vi "vision process goal.vi"(8 "Luma Range":cluster{"Lower value":i32, "Upper value":i32}={"Lower value"=40, "Upper value"=255}, 9 "Sat Range":cluster{"Lower value":i32, "Upper value":i32}={"Lower value"=52, "Upper value"=255}, 10 "Hue Range":cluster{"Lower value":i32, "Upper value":i32}={"Lower value"=80, "Upper value"=120}, 11 "Src Image":T1(plugin-control)) -> (2 "Annotated Image Out":T1(plugin-control), 3 "Processed Image Out":T1(plugin-control), 4 "Waveform Chart":dbl(graph))   [LabVIEW 2015]
uses:
  <vilib>/Rock Robotics/Network Tables/NT Read Boolean.vi
  <vilib>/Rock Robotics/Network Tables/NT Write Boolean.vi
  <vilib>/Rock Robotics/Network Tables/NT Write Number.vi
  <vilib>/vision/NI_Vision_Development_Module.lvlib
panel:
  out "output cluster":cluster{dbl[], dbl[], dbl[]}
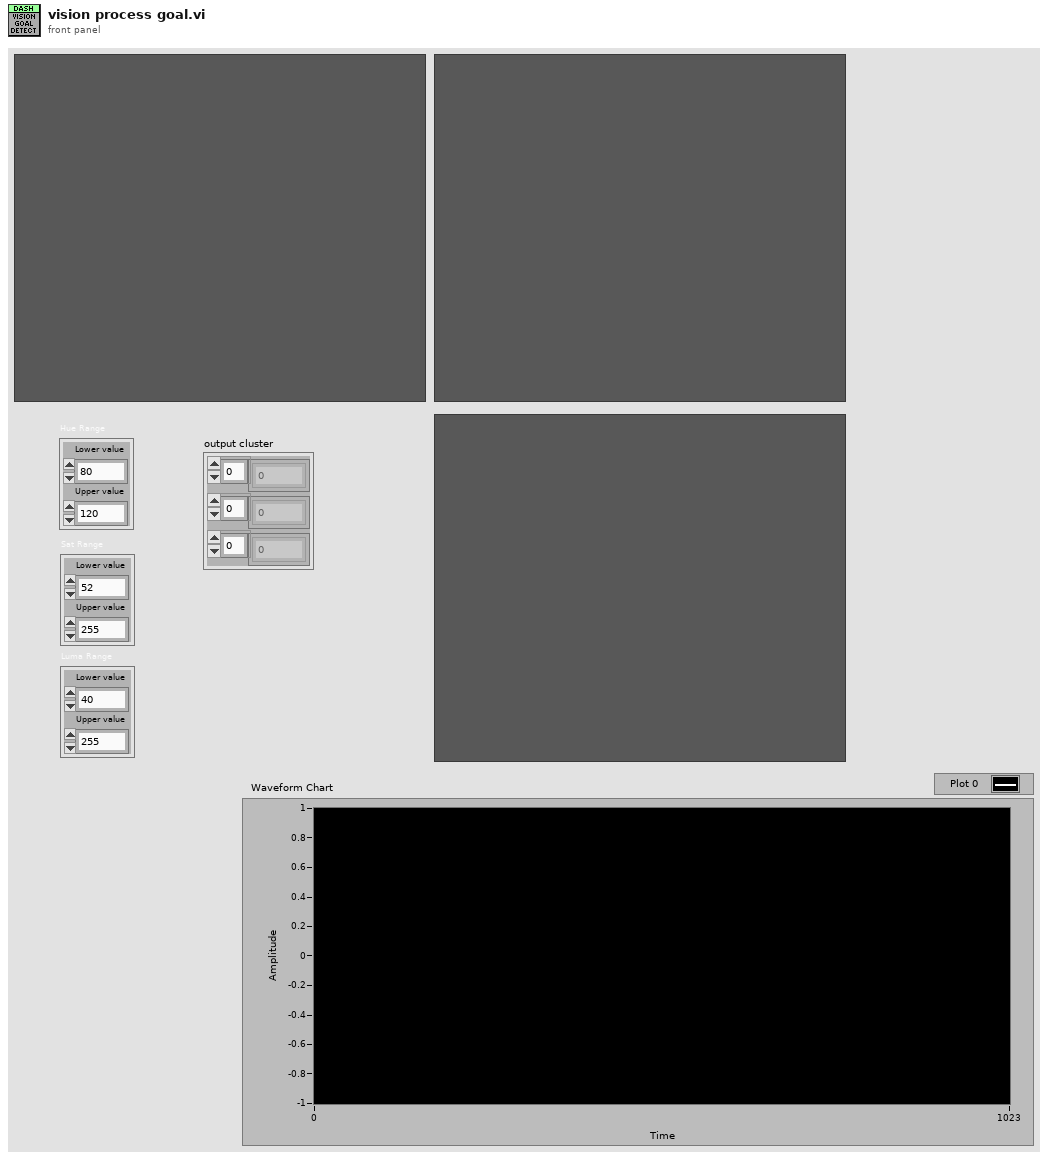
[diagram p1: front panel]
types:
  T1 = typedef "IMAQ Image.ctl" = refnum<image>
  T2 = typedef "Image Type" = u32
  T3 = cluster{"Area":dbl, "Number of Holes":dbl, "Bounding Rect":cluster{"Left":dbl, "Top":dbl, "Right":dbl, "Bottom":dbl}, "Center of Mass":cluster{"X":dbl, "Y":dbl}, "Orientation":dbl, "Dimensions":cluster{"Width":dbl, "Height":dbl}}
  T4 = cluster{"Desired Font (Application)":enum16{"User-specified Font", "Application Font", "System Font", "Dialog Font"}, "[User-specified Font]":cluster{"Font Name":string, "Size":i16, "Strikeout?":bool, "Italic?":bool, "Underline?":bool, "Outline?":bool, "Shadow?":bool, "Bold?":bool, "Rotation Angle":dbl}, "Horizontal Alignment":i16, "Vertical Alignment":i16}
  T5 = cluster{"Left":i32, "Top":i32, "Right":i32, "Bottom":i32}
  T6 = cluster{"Area":dbl, "Number of Holes":dbl, "Bounding Rect":cluster{"Left":dbl, "Top":dbl, "Right":dbl, "Bottom":dbl}, "Center of Mass":cluster{"X":dbl, "Y":dbl}, "Orientation":dbl, "Dimensions":cluster{"Width":dbl, "Height":dbl}}[]
  T7 = cluster{"Left":dbl, "Top":dbl, "Right":dbl, "Bottom":dbl}
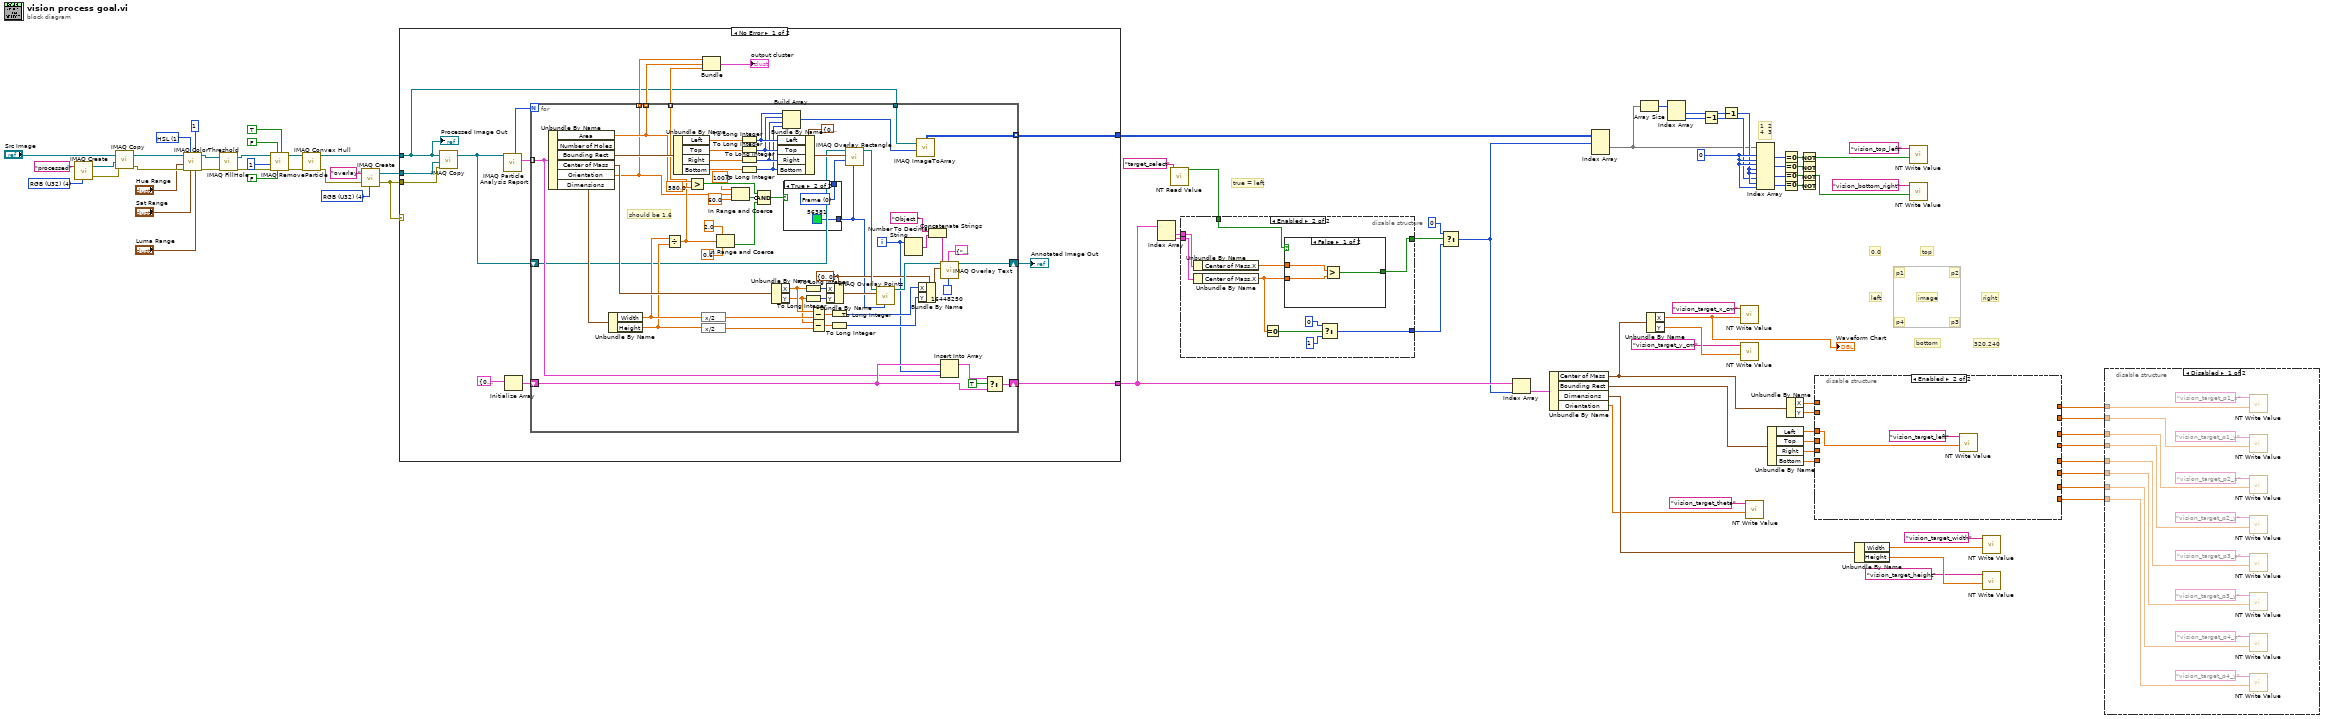
[diagram p0: block diagram]
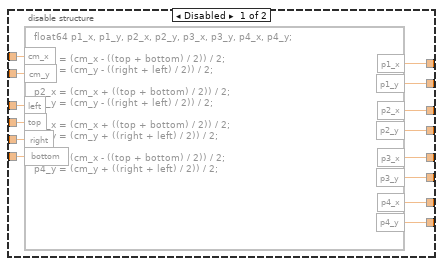
[diagram p3: hidden frame]
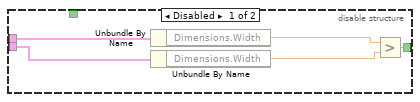
[diagram p4: hidden frame]
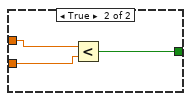
[diagram p5: hidden frame]
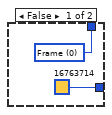
[diagram p6: hidden frame]
diagram:
  w36 = 0 ("index (row)")
  w77 = u16 1 items=["RGB", "HSL", "HSV", "HSI"] ("Color Mode")
  w79 = T2 4 items=["Grayscale (U8)", "Grayscale (I16)", "Grayscale (SGL)", "Complex (CSG)", "RGB (U32)", "HSL (U32)", "RGB (U64)", "Grayscale (U16)"] ("Image Type")
  w83 = T2 4 items=["Grayscale (U8)", "Grayscale (I16)", "Grayscale (SGL)", "Complex (CSG)", "RGB (U32)", "HSL (U32)", "RGB (U64)", "Grayscale (U16)"] ("Image Type")
  # "true = left"
  # "1  2\n4  3"
  # "320,240"
  # "0,0"
  # "top"
  # "right"
  # "left"
  # "bottom"
  # "image"
  # "p4"
  # "p3"
  # "p2"
  # "p1"
  n1 = call "IMAQ Create"("Image Name"="processed", "Image Type"=w79) -> ("New Image"=w80:T1, "error out"=w78:errorcluster)  [unwired: 3 in]
  n2 = call "IMAQ Copy"("error in (no error)"=w78, "Image Dst"=w80, "Image Src"="Src Image") -> ("error out"=w62:errorcluster, "Image Dst Out"=w73:T1)  [unwired: 3 in]
  n3 = call "IMAQ ColorThreshold"("Blue or Luma or Val or Inten Range"="Luma Range", "Replace Value"=1, "Green or Sat Range"="Sat Range", "Color Mode"=w77, "error in (no error)"=w62, "Red or Hue Range"="Hue Range", "Image Src"=w73) -> ("error out"=w63:errorcluster, "Image Dst Out"=w74:T1)  [unwired: 3 in]
  n4 = call "IMAQ FillHole"("error in (no error)"=w63, "Image Src"=w74) -> ("error out"=w64:errorcluster, "Image Dst Out"=w71:T1)  [unwired: 4 in]
  n5 = call "IMAQ RemoveParticle"("Connectivity 4/8 (8)"=TRUE, "Low Pass/High Pass (Low)"=FALSE, "Square/Hexa (Square)"=FALSE, "error in (no error)"=w64, "Number of Erosion"=1, "Image Src"=w71) -> ("error out"=w65:errorcluster, "Image Dst Out"=w66:T1)  [unwired: 1 in, 3 out]
  n6 = call "IMAQ Convex Hull"("error in (no error)"=w65, "Image Src"=w66) -> ("error out"=w58:errorcluster, "Image Dst Out"=w59:T1)  [unwired: 8 in]
  n7 = call "IMAQ Create"("Image Name"="overlay", "Image Type"=w83, "error in (no error)"=w58) -> ("New Image"=w84:T1, "error out"=w82:errorcluster)  [unwired: 2 in]
  n8 = case shown="No Error" w82 {
    tunnel: w84 -> [w97 _]
    tunnel: w59 -> [w86 _]
    tunnel: w82 -> [w96 _]
    tunnel: [w89 _] -> w12
    tunnel: [w88 _] -> w57
    frame No Error {
      n9 = call "IMAQ Copy"("error in (no error)"=w96, "Image Dst"=w97, "Image Src"=w86) -> ("Image Dst Out"=w87:T1)  [unwired: 3 in, 1 out]
      n10 = call "IMAQ Particle Analysis Report"("Image"=w87) -> ("Particle Reports (Pixels)"=w99:T6, "Number of Particles"=w100:i32)  [unwired: 5 in, 4 out]
      n11 = Initialize Array(T3 {"Area"=0.0, "Number of Holes"=0.0, "Bounding Rect"={"Left"=0.0, "Top"=0.0, "Right"=0.0, "Bottom"=0.0}, "Center of Mass"={"X"=0.0, "Y"=0.0}, "Orientation"=0.0, "Dimensions"={"Width"=0.0, "Height"=0.0}} ("Particle Report")) -> (w90:T6)  [unwired: 1 in]
      n12 = for {
        N: w100 -> [_]
        tunnel: w99 -> [w112] mode=indexing
        shift-right: [w147] -> w98
        shift-left: w87 -> [w110]
        tunnel: [w117] -> w95 mode=indexing
        tunnel: [w120] -> w94 mode=indexing
        tunnel: [w119] -> w93 mode=indexing
        shift-right: [w114] -> w89
        shift-left: w90 -> [w113]
        tunnel: [w103] -> w88 mode=indexing
        tunnel: w86 -> [w105]
        i -> [w101]
        w141 = cluster{"X":i32, "Y":i32} {"X"=0, "Y"=0} ("Point")
        # "should be 1.6"
        n13 = Unbundle By Name(w112) -> ("Area"=w120:dbl, "Bounding Rect"=w159:T7, "Center of Mass"=w153:cluster{"X":dbl, "Y":dbl}, "Orientation"=w117:dbl, "Dimensions"=w140:cluster{"Width":dbl, "Height":dbl})  [unwired: 1 out]
        n14 = Unbundle By Name(w140) -> ("Width"=w132:dbl, "Height"=w131:dbl)
        n15 = Divide(x=w132, y=w131) -> (x/y=w119:dbl)
        n16 = Unbundle By Name(w159) -> ("Left"=w157:dbl, "Top"=w156:dbl, "Right"=w155:dbl, "Bottom"=w125:dbl)
        n17 = Greater?(x=w120, y=580.0) -> (0:w123:bool)
        n18 = expression code="x/2"(w132) -> (w139:dbl)
        n19 = expression code="x/2"(w131) -> (w135:dbl)
        n20 = In Range and Coerce(upper limit=2.0, x=w119, lower limit=0.6 ("upper limit")) -> (In Range?=w128:bool)  [unwired: 1 out]
        n21 = In Range and Coerce(upper limit=100.0, x=w117, lower limit=60.0 ("y")) -> (In Range?=w118:bool)  [unwired: 1 out]
        n22 = To Long Integer(number=w157) -> (32bit integer=w109:i32)
        n23 = To Long Integer(number=w156) -> (32bit integer=w108:i32)
        n24 = To Long Integer(number=w155) -> (32bit integer=w107:i32)
        n25 = To Long Integer(number=w125) -> (32bit integer=w106:i32)
        n26 = Compound Arithmetic op=AND(w123, invert w118, w128) -> (w104:bool)
        n27 = Unbundle By Name(w153) -> ("X"=w122:dbl, "Y"=w121:dbl)
        n28 = Bundle By Name(cluster=T5 {"Left"=0, "Top"=0, "Right"=0, "Bottom"=0} ("Rectangle"), "Left"=w109, "Top"=w108, "Right"=w107, "Bottom"=w106) -> (w154:T5)
        n29 = Build Array(w109, w108, w107, w106) -> (w102:i32[])
        n30 = case shown="True" w104 {
          tunnel: [u32 16763714 ("Color") u32 56381 ("Color")] -> w127
          tunnel: [w161 w163] -> w126
          frame False {
            w161 = u32 0 items=["Frame", "Fill", "Highlight"] ("Drawing Mode (Frame)")
          }
          frame True {
            w163 = u32 0 items=["Frame", "Fill", "Highlight"] ("Drawing Mode (Frame)")
          }
        }
        n31 = To Long Integer(number=w122) -> (32bit integer=w151:i32)
        n32 = To Long Integer(number=w121) -> (32bit integer=w152:i32)
        n33 = Subtract(x=w122, y=w139) -> (x-y=w138:dbl)
        n34 = Subtract(x=w121, y=w135) -> (x-y=w136:dbl)
        n35 = Bundle By Name(cluster=w141, "X"=w151, "Y"=w152) -> (w150:cluster{"X":i32, "Y":i32})
        n36 = To Long Integer(number=w138) -> (32bit integer=w137:i32)
        n37 = To Long Integer(number=w136) -> (32bit integer=w134:i32)
        n38 = call "IMAQ Overlay Rectangle"("Color"=w127, "Drawing Mode (Frame)"=w126, "Rectangle"=w154, "Image"=w110) -> ("Image Out"=w149:T1)  [unwired: 6 in, 1 out]
        n39 = call "IMAQ Overlay Points"("Color"=w127, "Point"=w150, "Image"=w149) -> ("Image Out"=w148:T1)  [unwired: 7 in, 1 out]
        n40 = Number To Decimal String(number=w101) -> (decimal integer string=w144:string)  [unwired: 1 in]
        n41 = call "IMAQ ImageToArray"("Optional Rectangle"=w102, "Image"=w105) -> ("Image Pixels (U8)"=w103:u8[][])  [unwired: 2 in, 4 out]
        n42 = Bundle By Name(cluster=w141, "X"=w137, "Y"=w134) -> (w142:cluster{"X":i32, "Y":i32})
        n43 = Concatenate Strings("Object " ("String"), w144) -> (w143:string)
        n44 = call "IMAQ Overlay Text"("Text Color (black)"=u32 16448250 ("Color"), "Font, Size & Style"=T4 {"Desired Font (Application)"=enum."User-specified Font", "[User-specified Font]"={"Font Name"="Roboto Light", "Size"=12, "Strikeout?"=FALSE, "Italic?"=FALSE, "Underline?"=FALSE, "Outline?"=FALSE, "Shadow?"=FALSE, "Bold?"=FALSE, "Rotation Angle"=0.0}, "Horizontal Alignment"=0, "Vertical Alignment"=0}, "String"=w143, "Origin"=w142, "Image"=w148) -> ("Image Out"=w147:T1)  [unwired: 5 in, 1 out]
        n45 = Insert Into Array(array=w113, index=w101, new element=w112) -> (w160:T6)
        n46 = Select(t=w160, s=TRUE, f=w113) -> (s? t:f=w114:T6)
      }
      "Annotated Image Out" <- w98
      n47 = Bundle(w95, w94, w93) -> (→"output cluster":cluster{dbl[], dbl[], dbl[]})  [unwired: 1 in]
      "Processed Image Out" <- w86
    }
    frame Error {
    }
  }
  n48 = Index Array(array=w12) -> (element #1=w11:T3, element #2=w10:T3)  [unwired: 2 in]
  n49 = call-poly <vilib>:"NT Read Value.vi"("Name"="target_select") -> ("Boolean"=w6:bool)  [unwired: 9 in, 1 out]
  n50 = disable-structure shown="Enabled" {
    disable-tunnel: w11 -> [w169 w179]
    disable-tunnel: w10 -> [w168 w178]
    disable-tunnel: w6 -> [_ w177]
    disable-tunnel: [w166 w175] -> w5
    disable-tunnel: [_ w170] -> w2
    frame Disabled {
      n51 = Unbundle By Name(w169) -> ("Dimensions.Width"=w165:dbl)
      n52 = Unbundle By Name(w168) -> ("Dimensions.Width"=w167:dbl)
      n53 = Greater?(x=w165, y=w167) -> (0:w166:bool)
    }
    frame Enabled {
      n54 = Unbundle By Name(w179) -> ("Center of Mass.X"=w176:dbl)
      n55 = Unbundle By Name(w178) -> ("Center of Mass.X"=w174:dbl)
      n56 = Equal To 0?(x=w174) -> (x = 0?=w173:bool)
      n57 = case shown="False" w177 {
        tunnel: w176 -> [w182 w185]
        tunnel: w174 -> [w181 w184]
        tunnel: [w180 w183] -> w175
        frame False {
          n58 = Greater?(x=w182, y=w181) -> (0:w180:bool)
        }
        frame True {
          n59 = Less?(x=w185, y=w184) -> (x < y?=w183:bool)
        }
      }
      n60 = Select(t=0, s=w173, f=1) -> (s? t:f=w170:i32)
    }
  }
  n61 = Select(t=0, s=w5, f=w2) -> (s? t:f=w8:i32)
  n62 = Index Array(array=w12, index=w8) -> (element=w39:T3)
  n63 = Unbundle By Name(w39) -> ("Center of Mass"=w49:cluster{"X":dbl, "Y":dbl}, "Bounding Rect"=w50:T7, "Dimensions"=w48:cluster{"Width":dbl, "Height":dbl}, "Orientation"=w3:dbl)
  n64 = Index Array(array=w57, index (dim 0)=w8) -> (element=w32:u8[][])  [unwired: 2 in]
  n65 = Array Size(array=w32) -> (size(s)=w38:i32[])
  n66 = Unbundle By Name(w49) -> ("X"=w1:dbl, "Y"=w51:dbl)
  "Waveform Chart" <- w1
  n67 = Index Array(array=w38) -> (element #1=w35:i32, element #2=w37:i32)  [unwired: 2 in]
  n68 = Decrement(x=w37) -> (x-1=w33:i32)
  n69 = Decrement(x=w35) -> (x-1=w34:i32)
  n70 = call-poly <vilib>:"NT Write Value.vi"("Numeric"=w1, "Name"="vision_target_x_cm") -> ()  [unwired: 9 in, 1 out]
  n71 = call-poly <vilib>:"NT Write Value.vi"("Numeric"=w51, "Name"="vision_target_y_cm") -> ()  [unwired: 9 in, 1 out]
  n72 = call-poly <vilib>:"NT Write Value.vi"("Numeric"=w3, "Name"="vision_target_theta") -> ()  [unwired: 9 in, 1 out]
  n73 = Index Array(array=w32, index (row) #1=w36, index (col) #1=w36, index (row) #2=w36, index (col) #2=w34, index (row) #3=w34, index (col) #3=w33, index (row) #4=w34, index (col) #4=w36) -> (element #1=w31:u8, element #2=w30:u8, element #3=w29:u8, element #4=w28:u8)
  n74 = Unbundle By Name(w50) -> ("Left"=w21:dbl, "Top"=w20:dbl, "Right"=w19:dbl, "Bottom"=w18:dbl)
  n75 = Equal To 0?(x=w31) -> (x = 0?=w27:bool)
  n76 = Equal To 0?(x=w30) -> (x = 0?=w26:bool)
  n77 = Equal To 0?(x=w29) -> (x = 0?=w25:bool)
  n78 = Equal To 0?(x=w28) -> (x = 0?=w24:bool)
  n79 = Unbundle By Name(w49) -> ("X"=w23:dbl, "Y"=w22:dbl)
  n80 = Not(x=w27) -> (.not. x?=w13:bool)
  n81 = Not(x=w26) -> ()  [unwired: 1 out]
  n82 = Not(x=w25) -> (.not. x?=w14:bool)
  n83 = Not(x=w24) -> ()  [unwired: 1 out]
  n84 = disable-structure shown="Enabled" {
    disable-tunnel: [w199 _] -> w47
    disable-tunnel: [w198 _] -> w46
    disable-tunnel: [w197 _] -> w45
    disable-tunnel: [w196 _] -> w44
    disable-tunnel: [w195 _] -> w43
    disable-tunnel: [w194 _] -> w42
    disable-tunnel: [w193 _] -> w41
    disable-tunnel: w23 -> [w192 _]
    disable-tunnel: w22 -> [w191 _]
    disable-tunnel: w21 -> [w190 w200]
    disable-tunnel: w20 -> [w189 _]
    disable-tunnel: w19 -> [w188 _]
    disable-tunnel: w18 -> [w187 _]
    disable-tunnel: [w186 _] -> w17
    frame Disabled {
      n85 = formula code="float64 p1_x, p1_y, p2_x, p2_y, p3_x, p3_y, p4_x, p4_y;\n\np1_x = (cm_x - ((top + bottom) / 2)) / 2;\np1_y = (cm_y - ((right + left) / 2)) / 2;\n\np2_x = (cm_x + ((top + bottom) / 2)) / 2;\np2_y = (cm_y - ((right + left) / 2)) / 2;\n\np3_x = (cm_x + ((top + bottom) / 2)) / 2;\np3_y = (cm_y + ((right + left) / 2)) / 2;\n\np4_x = (cm_x - ((top + bottom) / 2)) / 2;\np4_y = (cm_y + ((right + left) / 2)) / 2;"("cm_x"=w192, "cm_y"=w191, "left"=w190, "top"=w189, "right"=w188, "bottom"=w187) -> ("p1_x"=w199:dbl, "p1_y"=w186:dbl, "p2_x"=w198:dbl, "p2_y"=w197:dbl, "p3_x"=w196:dbl, "p3_y"=w195:dbl, "p4_x"=w194:dbl, "p4_y"=w193:dbl)
    }
    frame Enabled {
      n86 = call-poly <vilib>:"NT Write Value.vi"("Numeric"=w200, "Name"="vision_target_left") -> ()  [unwired: 9 in, 1 out]
    }
  }
  n87 = Unbundle By Name(w48) -> ("Width"=w56:dbl, "Height"=w55:dbl)
  n88 = call-poly <vilib>:"NT Write Value.vi"("Boolean"=w13, "Name"="vision_top_left") -> ()  [unwired: 9 in, 1 out]
  n89 = call-poly <vilib>:"NT Write Value.vi"("Boolean"=w14, "Name"="vision_bottom_right") -> ()  [unwired: 9 in, 1 out]
  n90 = call-poly <vilib>:"NT Write Value.vi"("Numeric"=w56, "Name"="vision_target_width") -> ()  [unwired: 9 in, 1 out]
  n91 = call-poly <vilib>:"NT Write Value.vi"("Numeric"=w55, "Name"="vision_target_height") -> ()  [unwired: 9 in, 1 out]
  n92 = disable-structure shown="Disabled" {
    disable-tunnel: w47 -> [w217 _]
    disable-tunnel: w46 -> [w216 _]
    disable-tunnel: w45 -> [w215 _]
    disable-tunnel: w44 -> [w214 _]
    disable-tunnel: w43 -> [w213 _]
    disable-tunnel: w42 -> [w212 _]
    disable-tunnel: w41 -> [w211 _]
    disable-tunnel: w17 -> [w210 _]
    frame Disabled {
      n93 = call-poly <vilib>:"NT Write Value.vi"("Numeric"=w217, "Name"="vision_target_p1_x") -> ()  [unwired: 9 in, 1 out]
      n94 = call-poly <vilib>:"NT Write Value.vi"("Numeric"=w210, "Name"="vision_target_p1_y") -> ()  [unwired: 9 in, 1 out]
      n95 = call-poly <vilib>:"NT Write Value.vi"("Numeric"=w216, "Name"="vision_target_p2_x") -> ()  [unwired: 9 in, 1 out]
      n96 = call-poly <vilib>:"NT Write Value.vi"("Numeric"=w215, "Name"="vision_target_p2_y") -> ()  [unwired: 9 in, 1 out]
      n97 = call-poly <vilib>:"NT Write Value.vi"("Numeric"=w214, "Name"="vision_target_p3_x") -> ()  [unwired: 9 in, 1 out]
      n98 = call-poly <vilib>:"NT Write Value.vi"("Numeric"=w213, "Name"="vision_target_p3_y") -> ()  [unwired: 9 in, 1 out]
      n99 = call-poly <vilib>:"NT Write Value.vi"("Numeric"=w212, "Name"="vision_target_p4_x") -> ()  [unwired: 9 in, 1 out]
      n100 = call-poly <vilib>:"NT Write Value.vi"("Numeric"=w211, "Name"="vision_target_p4_y") -> ()  [unwired: 9 in, 1 out]
    }
    frame Enabled {
    }
  }
